vi "Dialog Box and Enter key.vi"(8 "milliseconds to wait":u32=5000, 11 "message":string="Hello World") -> ()   [LabVIEW 2013]
uses:
  user32.dll
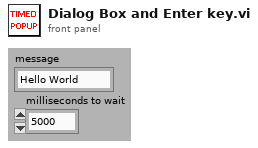
[diagram p1: front panel]
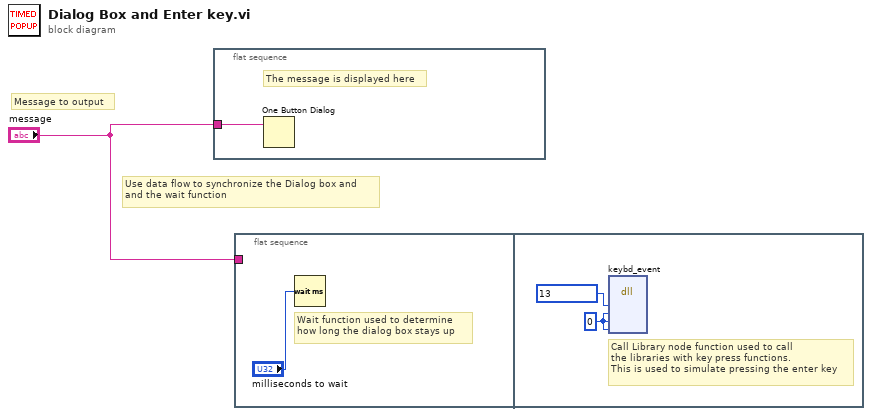
[diagram p0: block diagram]
diagram:
  # "Use data flow to synchronize the Dialog box and\nand the wait function"
  # "Message to output"
  n1 = flat-sequence {
    tunnel: "message" -> [w2]
    frame #0 {
      # "The message is displayed here"
      n2 = One Button Dialog(message=w2) -> ()  [unwired: 1 in, 1 out]
    }
  }
  n3 = flat-sequence {
    tunnel: "message" -> [_]
    frame #0 {
      # "Wait function used to determine \nhow long the dialog box stays up"
      n4 = Wait (ms)(milliseconds to wait="milliseconds to wait") -> ()  [unwired: 1 out]
    }
    frame #1 {
      w4 = u8 0 ("bScan")
      # "Call Library node function used to call \nthe libraries with key press functions. \nThis is used to simulate pressing the enter key"
      n5 = dll-call lib="user32.dll" fn="keybd_event"("bVk"=u8 13 ("Virtual Key"), "bScan"=w4, "dwFlags"=w4, "dwExtraInfo"=w4) -> ()  [unwired: 8 in, 2 out]
    }
  }
